vi "SEND_ABCPor.vi"(1 "设备地址 1 开始":i32) -> (0 "输出字符串":string)   [LabVIEW 2018]
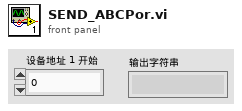
[diagram p1: front panel]
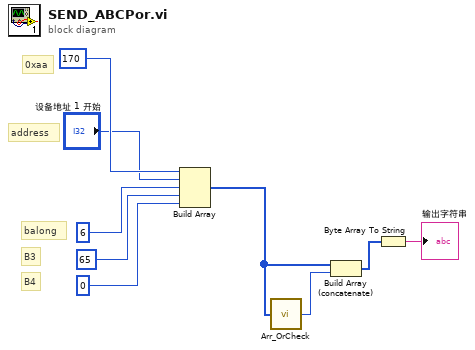
[diagram p0: block diagram]
diagram:
  # "B4"
  # "B3"
  # "balong"
  # "address"
  # "0xaa"
  n1 = Build Array(170, "设备地址 1 开始", 6, 65, 0) -> (w3:i32[])
  n2 = call "Arr_OrCheck.vi"("数组"=w3) -> ("抑或的数据值"=w9:u8)
  n3 = Build Array (concatenate)(w3, w9) -> (w8:i32[])
  n4 = Byte Array To String(unsigned byte array=w8) -> (string=→"输出字符串":string)
